vi "test ut fftw.vi"() -> ()   [LabVIEW 2014]
uses:
  <vilib>/Analysis/2dsp.llb/Real FFT.vi
  init.vi
  transform.vi
  cleanup.vi
  <vilib>/Analysis/NI_AALPro.lvlib
panel:
  out "FFTW Size":i32[](array[numeric])
  out "Labview Time":dbl
  out "CPP Time":dbl
  out "Intensity Graph":sgl[][](graph)
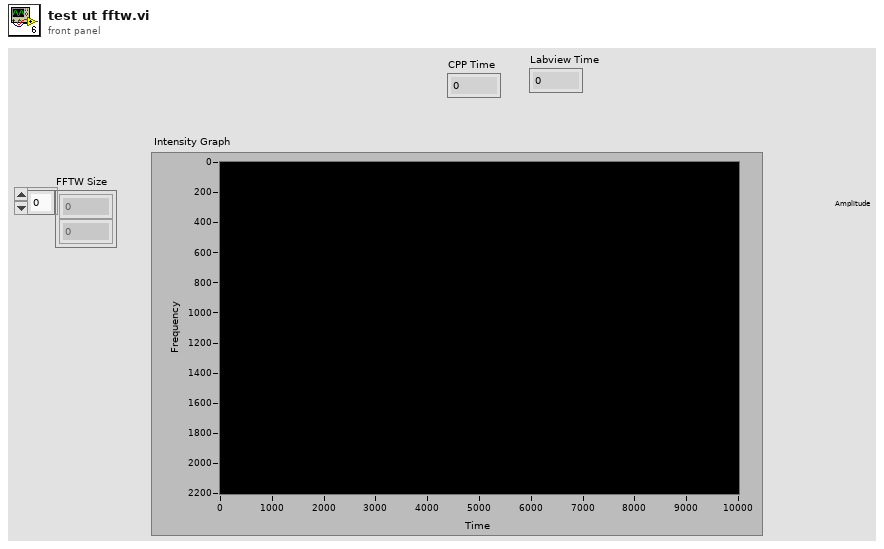
[diagram p1: front panel]
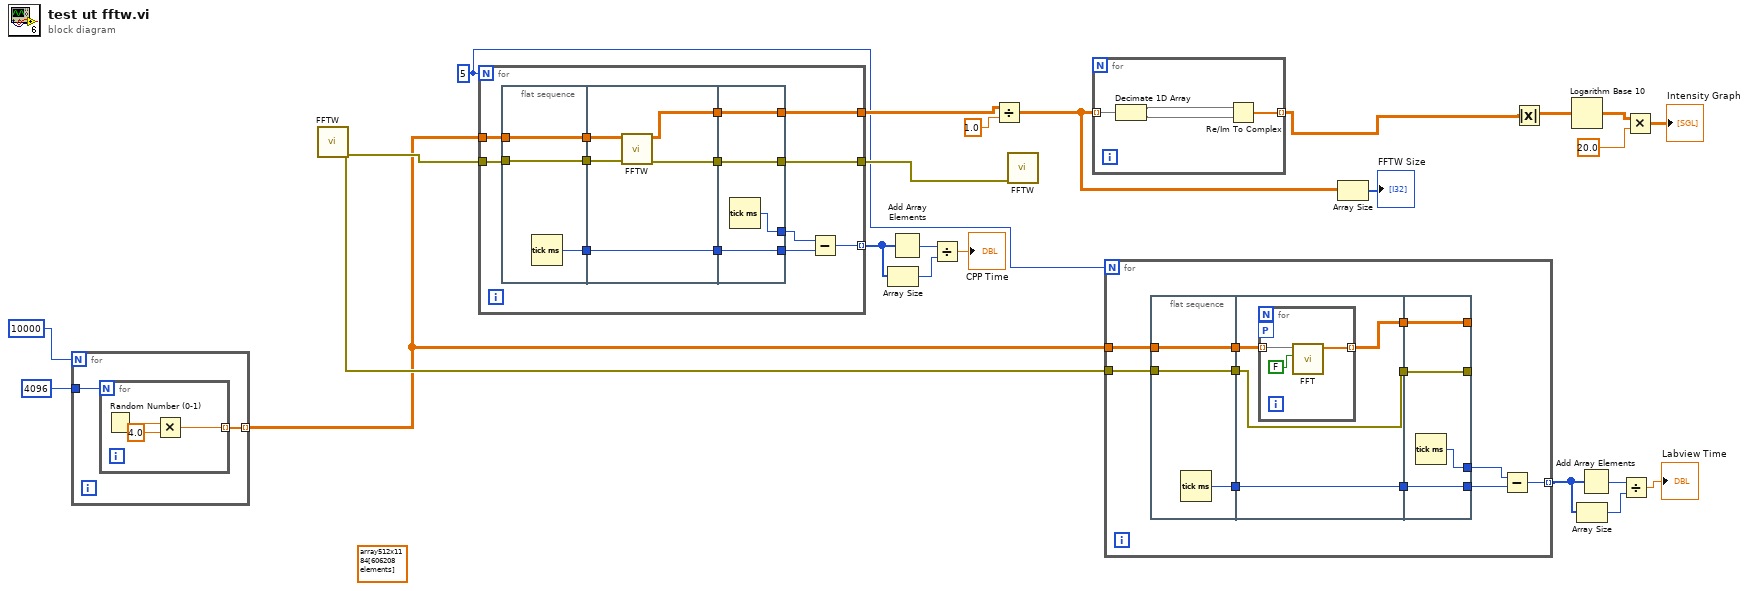
[diagram p0: block diagram]
diagram:
  w4 = 5
  (unwired) sgl[][] array512x1184[606208 elements]
  n1 = for {
    N: 10000 -> [_]
    tunnel: [w25] -> w3 mode=indexing
    tunnel: 4096 -> [w24]
    n2 = for {
      N: w24 -> [_]
      tunnel: [w26] -> w25 mode=indexing
      n3 = Random Number (0-1)() -> (number: 0 to 1=w28:dbl)
      n4 = Multiply(x=w28, y=4.0) -> (x*y=w26:dbl)
    }
  }
  n5 = call-poly "FFTW.vi"() -> ("Error Out"=w22:errorcluster)  [unwired: 11 in]
  n6 = for {
    N: w4 -> [_]
    tunnel: [w31] -> w15
    tunnel: w3 -> [w30]
    tunnel: [w29] -> w11 mode=indexing
    tunnel: w22 -> [w33]
    tunnel: [w35] -> w23
    n7 = flat-sequence {
      tunnel: w33 -> [w44]
      tunnel: w30 -> [w42]
      tunnel: [w42] -> w41
      tunnel: [w44] -> w40
      tunnel: [w43] -> w39
      tunnel: [w47] -> w38
      tunnel: [w46] -> w37
      tunnel: w41 -> [w49]
      tunnel: w40 -> [w48]
      tunnel: w39 -> [w45]
      tunnel: [w45] -> w36
      tunnel: [w52] -> w31
      tunnel: [w53] -> w35
      tunnel: w38 -> [w53]
      tunnel: w37 -> [w52]
      tunnel: [w51] -> w34
      tunnel: w36 -> [w50]
      tunnel: [w50] -> w32
      frame #0 {
        n8 = Tick Count (ms)() -> (millisecond timer value=w43:u32)
      }
      frame #1 {
        n9 = call-poly "FFTW.vi"("Error In"=w48, "Input"=w49) -> ("Error Out"=w47:errorcluster, "Output"=w46:sgl[][])  [unwired: 8 in]
      }
      frame #2 {
        n10 = Tick Count (ms)() -> (millisecond timer value=w51:u32)
      }
    }
    n11 = Subtract(x=w34, y=w32) -> (x-y=w29:u32)
  }
  n12 = Array Size(array=w11) -> (size(s)=w10:i32)
  n13 = Add Array Elements(numeric array=w11) -> (sum=w12:u32)
  n14 = Divide(x=w12, y=w10) -> (x/y=→"CPP Time":dbl)
  n15 = Divide(x=w15, y=sgl 1.0 ("dimension size")) -> (x/y=w13:sgl[][])
  n16 = call-poly "FFTW.vi"("Error In"=w23) -> ()  [unwired: 10 in, 1 out]
  n17 = for {
    tunnel: w13 -> [w56] mode=indexing
    tunnel: [w57] -> w16 mode=indexing
    n18 = Decimate 1D Array(w56) -> (w55:sgl[], w54:sgl[])
    n19 = Re/Im To Complex(1:w54, 2:w55) -> (0:w57:csg[])
  }
  n20 = for {
    N: w4 -> [_]
    tunnel: w22 -> [w62]
    tunnel: [w61] -> w5 mode=indexing
    tunnel: w3 -> [w58]
    n21 = flat-sequence {
      tunnel: w62 -> [w70]
      tunnel: w58 -> [w71]
      tunnel: [w71] -> w68
      tunnel: [w70] -> w67
      tunnel: [w69] -> w66
      tunnel: [w72] -> w65
      tunnel: w68 -> [w73]
      tunnel: w67 -> [w74]
      tunnel: w66 -> [w75]
      tunnel: [w75] -> w64
      tunnel: [w74] -> w63
      tunnel: [w81] -> _
      tunnel: [w82] -> _
      tunnel: w65 -> [w81]
      tunnel: [w80] -> w59
      tunnel: w64 -> [w79]
      tunnel: [w79] -> w60
      tunnel: w63 -> [w82]
      frame #0 {
        n22 = Tick Count (ms)() -> (millisecond timer value=w69:u32)
      }
      frame #1 {
        n23 = for {
          tunnel: w73 -> [w78] mode=indexing
          tunnel: [w77] -> w72 mode=indexing
          workers-P: _ -> [_]
          n24 = call-poly <vilib>:"FFT.vi"("shift?"=FALSE, "X"=w78) -> ("FFT {X}"=w77:cdb[])  [unwired: 8 in, 1 out]
        }
      }
      frame #2 {
        n25 = Tick Count (ms)() -> (millisecond timer value=w80:u32)
      }
    }
    n26 = Subtract(x=w59, y=w60) -> (x-y=w61:u32)
  }
  n27 = Array Size(array=w13) -> (size(s)=→"FFTW Size":i32[])
  n28 = Absolute Value(x=w16) -> (abs(x)=w19:sgl[][])
  n29 = Logarithm Base 10(1:w19) -> (0:w18:sgl[][])
  n30 = Array Size(array=w5) -> (size(s)=w8:i32)
  n31 = Add Array Elements(numeric array=w5) -> (sum=w7:u32)
  n32 = Divide(x=w7, y=w8) -> (x/y=→"Labview Time":dbl)
  n33 = Multiply(x=w18, y=sgl 20.0 ("dimension size")) -> (x*y=→"Intensity Graph":sgl[][])
